vi "LinePolyClip.vi"() -> ()   [LabVIEW 2014]
uses:
  TypeDefs/Point2D.ctl
  TypeDefs/Poly2D.ctl
panel:
  out "sorted array":T2(array[cluster])
  in  "Lines":T3
  in  "Polys":T3[](array[typedef])
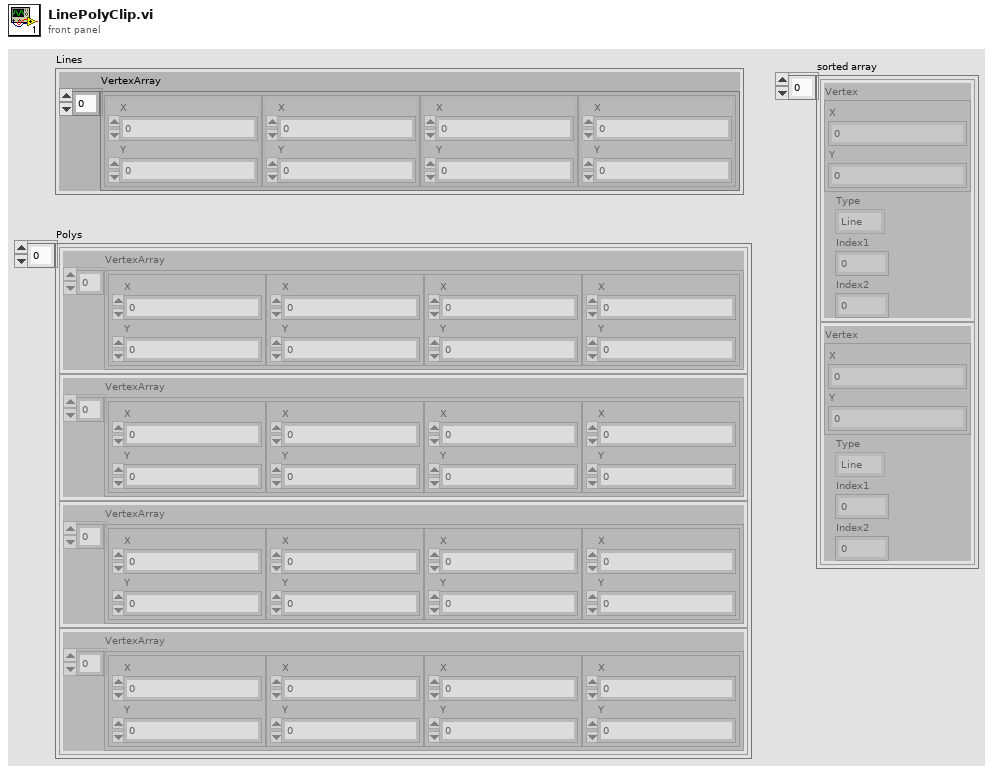
[diagram p1: front panel]
types:
  T1 = typedef "Point2D.ctl" = cluster{"X":sgl, "Y":sgl}
  T2 = cluster{"Vertex":T1, "Type":enum16{"Line", "Poly", "Cross"}, "Index1":i32, "Index2":i32}[]
  T3 = typedef "Poly2D.ctl" = cluster{"VertexArray":T1[]}
  T4 = cluster{"Line1":cluster{"Left":cluster{"Vertex":T1, "Type":enum16{"Line", "Poly", "Cross"}, "Index1":i32, "Index2":i32}, "Right":cluster{"Vertex":T1, "Type":enum16{"Line", "Poly", "Cross"}, "Index1":i32, "Index2":i32}}, "Line2":cluster{"Left":cluster{"Vertex":T1, "Type":enum16{"Line", "Poly", "Cross"}, "Index1":i32, "Index2":i32}, "Right":cluster{"Vertex":T1, "Type":enum16{"Line", "Poly", "Cross"}, "Index1":i32, "Index2":i32}}}[]
  T5 = cluster{"Left":cluster{"Vertex":T1, "Type":enum16{"Line", "Poly", "Cross"}, "Index1":i32, "Index2":i32}, "Right":cluster{"Vertex":T1, "Type":enum16{"Line", "Poly", "Cross"}, "Index1":i32, "Index2":i32}}[]
  T6 = cluster{"Vertex":T1, "Type":enum16{"Line", "Poly", "Cross"}, "Index1":i32, "Index2":i32}
  T7 = cluster{"Event":cluster{"Left":cluster{"Vertex":T1, "Type":enum16{"Line", "Poly", "Cross"}, "Index1":i32, "Index2":i32}, "Right":cluster{"Vertex":T1, "Type":enum16{"Line", "Poly", "Cross"}, "Index1":i32, "Index2":i32}}, "Operation":enum16{"Insert", "Delete"}}[]
  T8 = cluster{"Left":cluster{"Vertex":T1, "Type":enum16{"Line", "Poly", "Cross"}, "Index1":i32, "Index2":i32}, "Right":cluster{"Vertex":T1, "Type":enum16{"Line", "Poly", "Cross"}, "Index1":i32, "Index2":i32}}
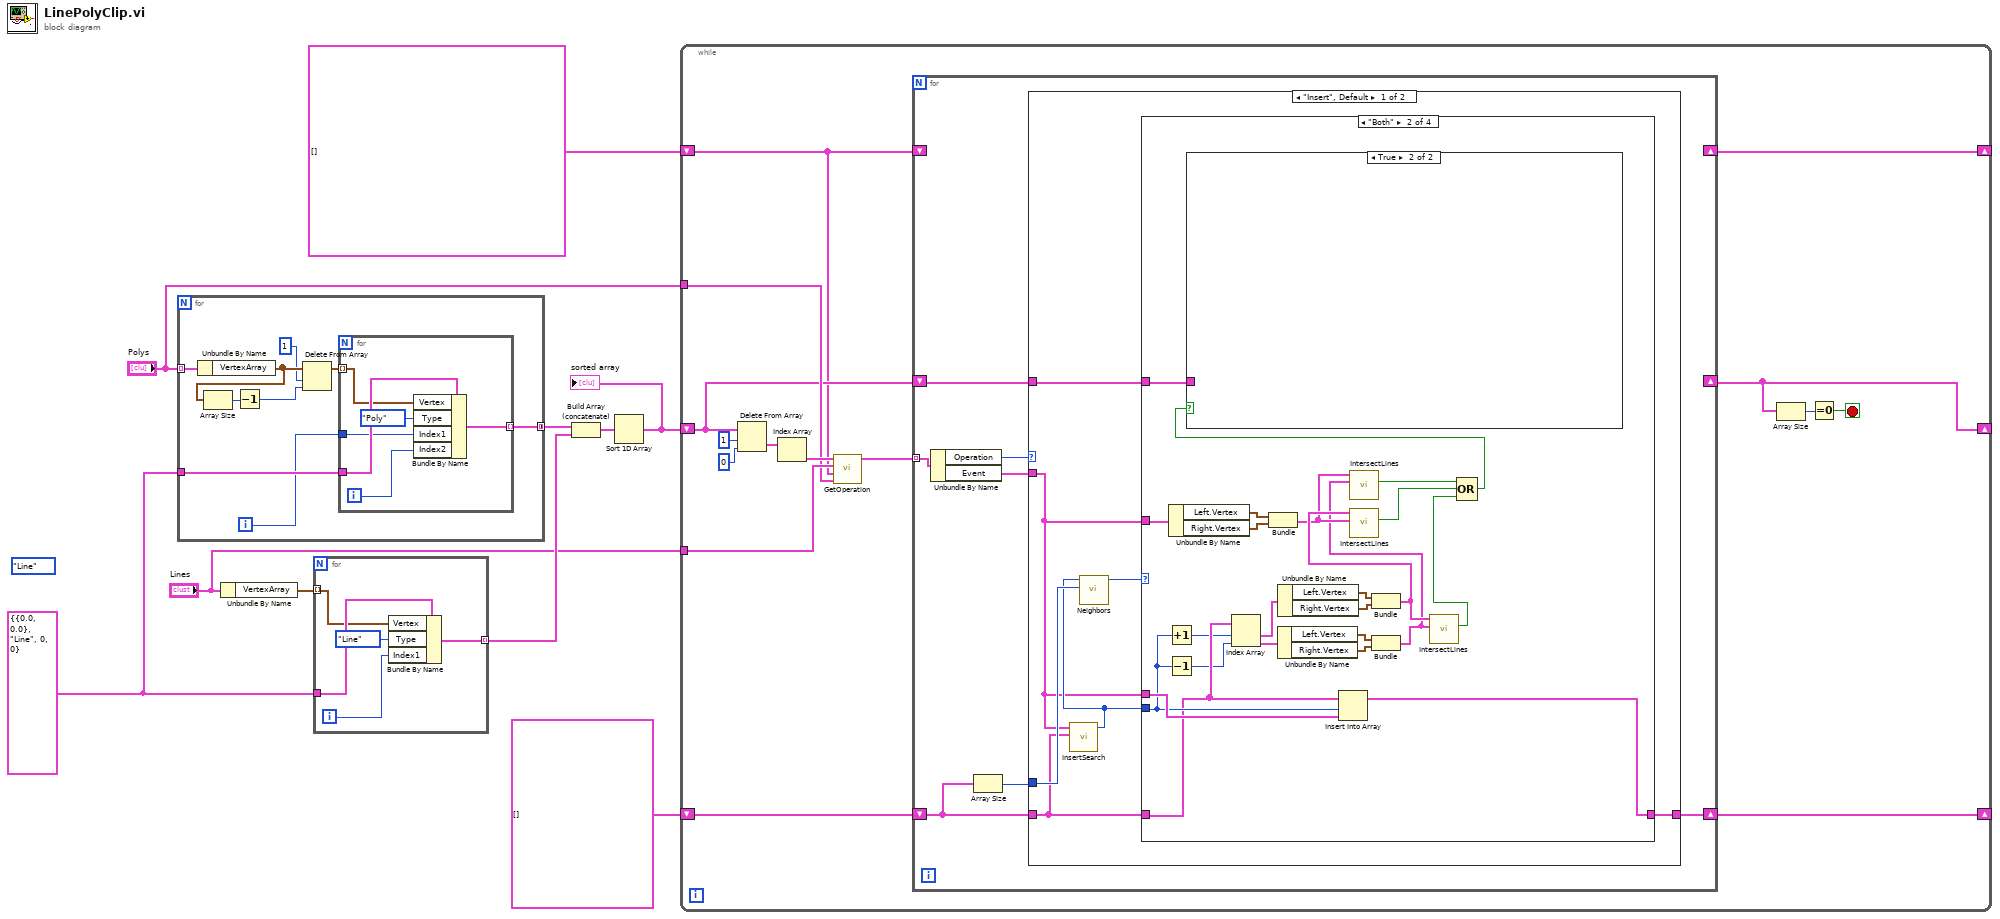
[diagram p0: block diagram]
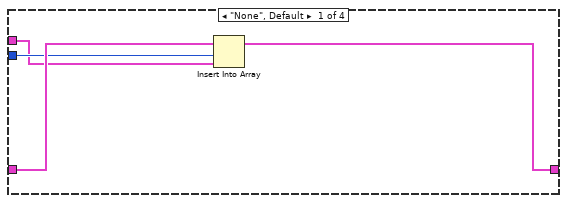
[diagram p2: hidden frame]
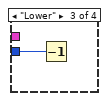
[diagram p4: hidden frame]
diagram:
  (unwired) enum16{"Line", "Poly", "Cross"}."Line"
  w9 = T6 {"Vertex"={"X"=0.0, "Y"=0.0}, "Type"=enum."Line", "Index1"=0, "Index2"=0}
  n1 = for {
    tunnel: "Polys" -> [w19] mode=indexing
    tunnel: w9 -> [w18]
    tunnel: [w16] -> w8 mode=concatenating
    i -> [w17]
    n2 = Unbundle By Name(w19) -> ("VertexArray"=w15:T1[])
    n3 = Array Size(array=w15) -> (size(s)=w12:i32)
    n4 = Decrement(x=w12) -> (x-1=w11:i32)
    n5 = Delete From Array(array=w15, length=1, index=w11) -> (array with subset deleted=w14:T1[])  [unwired: 1 out]
    n6 = for {
      tunnel: w14 -> [w24] mode=indexing
      tunnel: w18 -> [w25]
      tunnel: [w22] -> w16 mode=indexing
      tunnel: w17 -> [w21]
      i -> [w20]
      n7 = Bundle By Name(cluster=w25, "Vertex"=w24, "Type"=enum16{"Line", "Poly", "Cross"}."Poly", "Index1"=w21, "Index2"=w20) -> (w22:T6)
    }
  }
  n8 = Unbundle By Name("Lines") -> ("VertexArray"=w10:T1[])
  n9 = for {
    tunnel: w10 -> [w29] mode=indexing
    tunnel: w9 -> [w30]
    tunnel: [w26] -> w7 mode=indexing
    i -> [w27]
    n10 = Bundle By Name(cluster=w30, "Vertex"=w29, "Type"=enum16{"Line", "Poly", "Cross"}."Line", "Index1"=w27) -> (w26:T6)
  }
  n11 = Build Array (concatenate)(w8, w7) -> (w6:T2)
  n12 = Sort 1D Array(array=w6) -> (sorted array=w5:T2)
  "sorted array" <- w5
  n13 = while {
    shift-right: [w33] -> _
    shift-left: T5 [] -> [w37]
    shift-right: [w36] -> _
    shift-left: w5 -> [w38]
    shift-right: [w31] -> _
    shift-left: T4 [] -> [w32]
    tunnel: "Lines" -> [w41]
    tunnel: "Polys" -> [w40]
    stop <- w34 stop-if-true
    n14 = Delete From Array(array=w38, length=1, index=0) -> (deleted portion=w43:T2)  [unwired: 1 out]
    n15 = Index Array(array=w43) -> (element=w42:T6)  [unwired: 1 in]
    n16 = call "GetOperation.vi"("Polys"=w40, "Crossings"=w32, "Lines"=w41, "End"=w42) -> ("Operations"=w39:T7)  [unwired: 7 in]
    n17 = for {
      tunnel: w39 -> [w52] mode=indexing
      shift-right: [_] -> w36
      shift-left: w38 -> [w46]
      shift-right: [w47] -> w33
      shift-left: w37 -> [w49]
      shift-right: [_] -> w31
      shift-left: w32 -> [_]
      n18 = Unbundle By Name(w52) -> ("Operation"=w51:enum16{"Insert", "Delete"}, "Event"=w50:T8)
      n19 = Array Size(array=w49) -> (size(s)=w48:i32)
      n20 = case shown="\"Insert\", Default" w51 {
        tunnel: w49 -> [w57 _]
        tunnel: w50 -> [w54 _]
        tunnel: w48 -> [w59 _]
        tunnel: [w55 _] -> w47
        tunnel: w46 -> [w53 _]
        frame "Insert", Default {
          n21 = call "InsertSearch.vi"("EventQueue"=w57, "Event"=w54) -> ("Index"=w56:i32)  [unwired: 9 in]
          n22 = call "Neighbors.vi"("Size"=w59, "index"=w56) -> ("Neighbors"=w58:enum16{"None", "Both", "Lower", "Upper"})  [unwired: 9 in]
          n23 = case shown="\"Both\"" w58 {
            tunnel: w57 -> [w63 w83 _ _]
            tunnel: w56 -> [w62 w84 w87 _]
            tunnel: w54 -> [w61 w86 _ _]
            tunnel: [w60 w85 _ _] -> w55
            tunnel: w54 -> [_ w74 _ _]
            tunnel: w53 -> [_ w64 _ _]
            frame "None", Default {
              n24 = Insert Into Array(array=w63, index=w62, new element=w61) -> (w60:T5)
            }
            frame "Both" {
              n25 = Increment(x=w84) -> (x+1=w82:i32)
              n26 = Decrement(x=w84) -> (x-1=w81:i32)
              n27 = Unbundle By Name(w74) -> ("Left.Vertex"=w73:T1, "Right.Vertex"=w72:T1)
              n28 = Index Array(array=w83, index #1=w82, index #2=w81) -> (element #1=w80:T8, element #2=w77:T8)
              n29 = Bundle("Vertex"=w73, "Vertex"=w72) -> (w70:cluster{"Vertex":T1, "Vertex":T1})  [unwired: 1 in]
              n30 = Unbundle By Name(w77) -> ("Left.Vertex"=w76:T1, "Right.Vertex"=w75:T1)
              n31 = Unbundle By Name(w80) -> ("Left.Vertex"=w79:T1, "Right.Vertex"=w78:T1)
              n32 = Insert Into Array(array=w83, index=w84, new element=w86) -> (w85:T5)
              n33 = Bundle("Vertex"=w79, "Vertex"=w78) -> (w71:cluster{"Vertex":T1, "Vertex":T1})  [unwired: 1 in]
              n34 = call "IntersectLines.vi"("Line2D_2"=w70, "Line2D_1"=w71) -> ("Intersect?"=w67:bool)  [unwired: 8 in, 1 out]
              n35 = Bundle("Vertex"=w76, "Vertex"=w75) -> (w69:cluster{"Vertex":T1, "Vertex":T1})  [unwired: 1 in]
              n36 = call "IntersectLines.vi"("Line2D_2"=w69, "Line2D_1"=w70) -> ("Intersect?"=w68:bool)  [unwired: 8 in, 1 out]
              n37 = call "IntersectLines.vi"("Line2D_2"=w69, "Line2D_1"=w71) -> ("Intersect?"=w66:bool)  [unwired: 8 in, 1 out]
              n38 = Compound Arithmetic op=OR(w68, w67, w66) -> (w65:bool)
              n39 = case shown="True" w65 {
                tunnel: w64 -> [_ _]
                frame False {
                }
                frame True {
                }
              }
            }
            frame "Lower" {
              n40 = Decrement(x=w87) -> ()  [unwired: 1 out]
            }
            frame "Upper" {
            }
          }
        }
        frame "Delete" {
        }
      }
    }
    n41 = Array Size(array=w36) -> (size(s)=w35:i32)
    n42 = Equal To 0?(x=w35) -> (x = 0?=w34:bool)
  }
